vi "DER Randomize Statuses.vi"(10 "DeviceID":T2) -> (3 "DER_Status Array out":T1[](array[typedef]))   [LabVIEW 2018, in "IED Test Framework.lvlib" / "IED Test.lvclass"]
uses:
  IED Test.lvclass
  <vilib>/ORNL/CSEISMIC DDS/CSEISMIC DDS Base/Data Types/Controls/DeviceID.ctl
  <vilib>/ORNL/CSEISMIC DDS/CSEISMIC DDS Base/Data Types/DER_Status.ctl
  <vilib>/ORNL/CSEISMIC DDS/CSEISMIC DDS Base/Data Types/Controls/DroopCurve.ctl
  <vilib>/ORNL/CSEISMIC DDS/CSEISMIC DDS Base/CSEISMIC DDS.lvclass
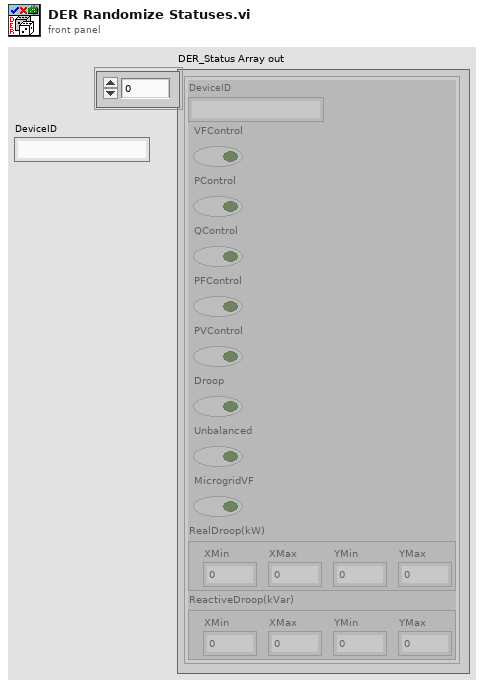
[diagram p1: front panel]
types:
  T1 = typedef "CSEISMIC DDS.lvlib/CSEISMIC DDS.lvclass/DER_Status.ctl" = cluster{"DeviceID":T2, "VFControl":bool, "PControl":bool, "QControl":bool, "PFControl":bool, "PVControl":bool, "Droop":bool, "Unbalanced":bool, "MicrogridVF":bool, "RealDroop(kW)":T3, "ReactiveDroop(kVar)":T3}
  T2 = typedef "CSEISMIC DDS.lvlib/CSEISMIC DDS.lvclass/DeviceID.ctl" = string
  T3 = typedef "CSEISMIC DDS.lvlib/CSEISMIC DDS.lvclass/DroopCurve.ctl" = cluster{"XMin":dbl, "XMax":dbl, "YMin":dbl, "YMax":dbl}
  T4 = cluster{"[0]":dbl, "[1]":dbl, "[2]":dbl, "[3]":dbl}
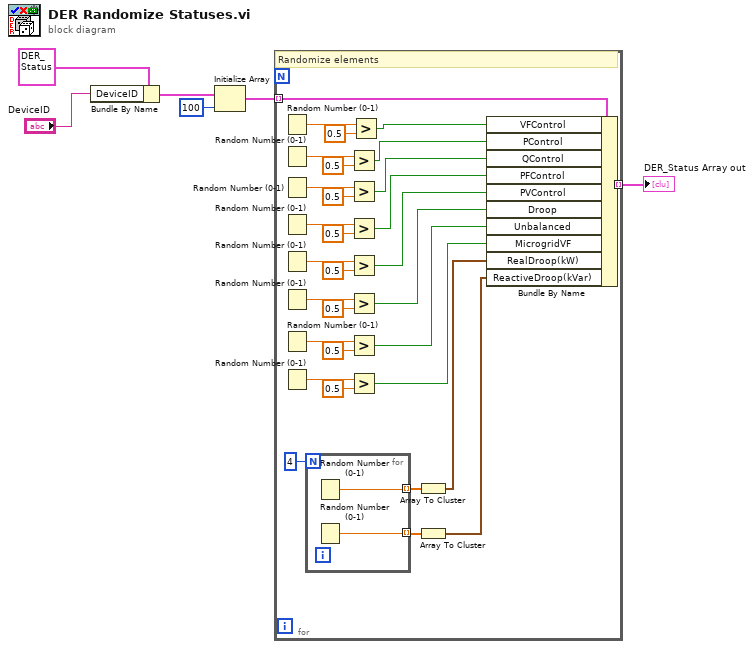
[diagram p0: block diagram]
diagram:
  n1 = Bundle By Name(cluster=T1 {"DeviceID"="", "VFControl"=FALSE, "PControl"=FALSE, "QControl"=FALSE, "PFControl"=FALSE, "PVControl"=FALSE, "Droop"=FALSE, "Unbalanced"=FALSE, "MicrogridVF"=FALSE, "RealDroop(kW)"={"XMin"=0.0, "XMax"=0.0, "YMin"=0.0, "YMax"=0.0}, "ReactiveDroop(kVar)"={"XMin"=0.0, "XMax"=0.0, "YMin"=0.0, "YMax"=0.0}} ("DER_Status"), "DeviceID"="DeviceID") -> (w5:T1)
  n2 = Initialize Array(w5, 100 ("dimension size")) -> (w2:T1[])
  n3 = for {
    tunnel: w2 -> [w37] mode=indexing
    tunnel: [w36] -> w1 mode=indexing
    # "Randomize elements"
    n4 = Random Number (0-1)() -> (number: 0 to 1=w35:dbl)
    n5 = Random Number (0-1)() -> (number: 0 to 1=w30:dbl)
    n6 = Random Number (0-1)() -> (number: 0 to 1=w29:dbl)
    n7 = Random Number (0-1)() -> (number: 0 to 1=w26:dbl)
    n8 = Random Number (0-1)() -> (number: 0 to 1=w23:dbl)
    n9 = Random Number (0-1)() -> (number: 0 to 1=w20:dbl)
    n10 = Random Number (0-1)() -> (number: 0 to 1=w15:dbl)
    n11 = Random Number (0-1)() -> (number: 0 to 1=w16:dbl)
    n12 = for {
      N: 4 -> [_]
      tunnel: [w39] -> w10 mode=indexing
      tunnel: [w38] -> w9 mode=indexing
      n13 = Random Number (0-1)() -> (number: 0 to 1=w39:dbl)
      n14 = Random Number (0-1)() -> (number: 0 to 1=w38:dbl)
    }
    n15 = Greater?(x=w30, y=0.5) -> (0:w28:bool)
    n16 = Greater?(x=w29, y=0.5) -> (0:w27:bool)
    n17 = Greater?(x=w26, y=0.5) -> (0:w22:bool)
    n18 = Greater?(x=w23, y=0.5) -> (0:w21:bool)
    n19 = Greater?(x=w20, y=0.5) -> (0:w18:bool)
    n20 = Greater?(x=w15, y=0.5) -> (0:w13:bool)
    n21 = Greater?(x=w16, y=0.5) -> (0:w12:bool)
    n22 = Greater?(x=w35, y=0.5) -> (0:w34:bool)
    n23 = Array To Cluster(array=w10) -> (cluster=w8:T4)
    n24 = Array To Cluster(array=w9) -> (cluster=w7:T4)
    n25 = Bundle By Name(cluster=w37, "VFControl"=w34, "PControl"=w28, "QControl"=w27, "PFControl"=w22, "PVControl"=w21, "Droop"=w18, "Unbalanced"=w13, "MicrogridVF"=w12, "RealDroop(kW)"=w8, "ReactiveDroop(kVar)"=w7) -> (w36:T1)
  }
  "DER_Status Array out" <- w1
